vi "simple_rag_qa_chat_agent.vi"() -> ()   [LabVIEW 2020]
uses:
  <userlib>/_Soliton/LabVIEW LLM Libraries/models/llm_openai_chatmodels/llm_openai_chatmodels.lvclass
  C:/Program Files/National Instruments/LabVIEW 2020/user.lib/_Soliton/LabVIEW LLM Libraries/models/abstract_llm_base/abstract_llm_base.lvclass
  <userlib>/_Soliton/LabVIEW LLM Libraries/vectorstore/vector_qdrant/vector_qdrant.lvclass
  C:/Program Files/National Instruments/LabVIEW 2020/user.lib/_Soliton/LabVIEW LLM Libraries/vectorstore/abstract_vector_base/abstract_vector_base.lvclass
  <userlib>/_Soliton/LabVIEW LLM Libraries/models/llm_openai_embedding/llm_openai_embedding.lvclass
  <userlib>/_Soliton/LabVIEW LLM Libraries/models/llm_openai_chatmodels/Instantiate_llm_openai.vi
  <userlib>/_Soliton/LabVIEW LLM Libraries/models/llm_openai_embedding/Instantiate_llm_openai_embed.vi
  <userlib>/_Soliton/LabVIEW LLM Libraries/models/message_text/create_text_message.vi
  <userlib>/_Soliton/LabVIEW LLM Libraries/agent/agent_simple_qa/agent_simple_qa.lvclass
  <userlib>/_Soliton/LabVIEW LLM Libraries/user_interfaces/simple_html_chat_ui/simple_html_chat_ui.lvclass
  <userlib>/_Soliton/LabVIEW LLM Libraries/models/message_text/message_text.lvclass
panel:
  in  "new_message":string
  in  "send":bool
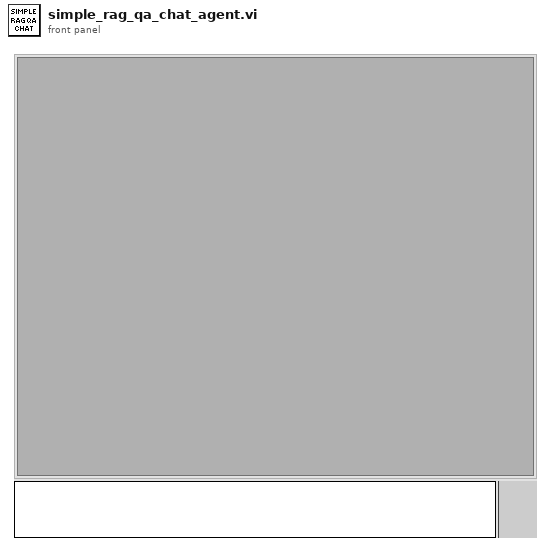
[diagram p1: front panel]
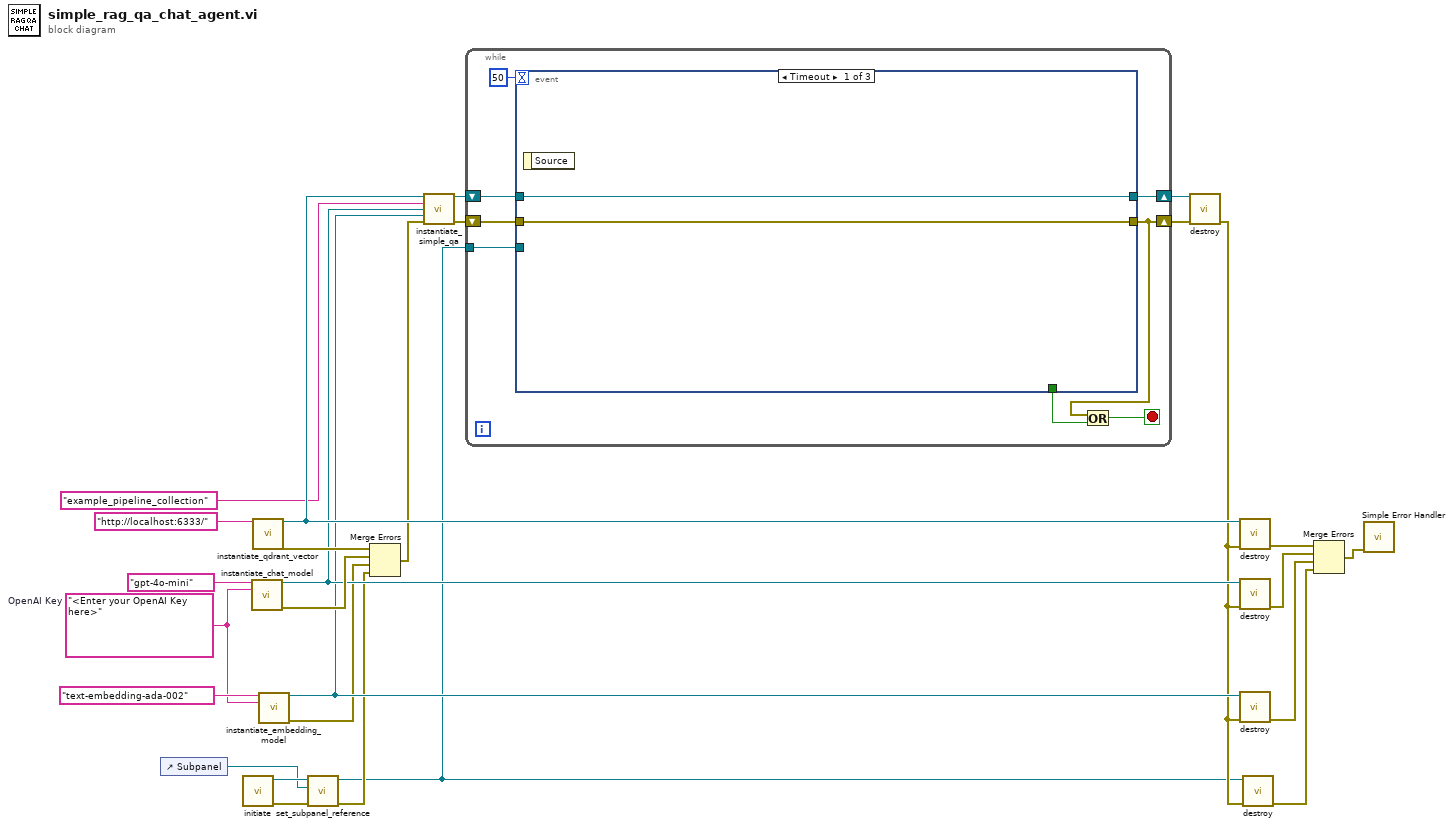
[diagram p0: block diagram]
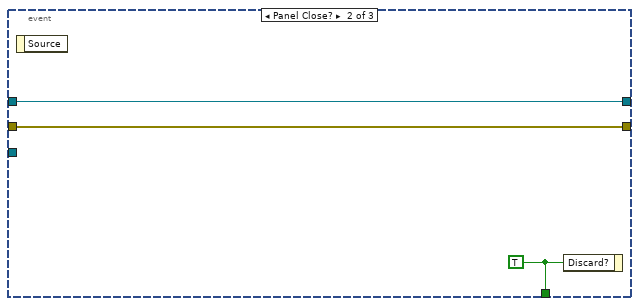
[diagram p2: hidden frame]
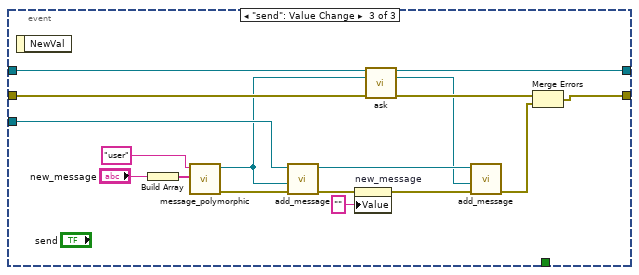
[diagram p3: hidden frame]
diagram:
  w1 = "<Enter your OpenAI Key here>"  # OpenAI Key
  n1 = control-ref of="Subpanel"() -> (w5:refnum<vi>)
  n2 = call <userlib>:"initiate.vi"() -> ("error out"=w8:errorcluster, "simple_html_chat_ui out"=w6:refnum<class "simple_html_chat_ui.lvclass">)  [unwired: 10 in]
  n3 = call-poly <userlib>:"instantiate_chat_model.vi"("model_name"="gpt-4o-mini", "openai_key"=w1) -> ("llm_openai out"=w14:refnum<class "llm_openai_chatmodels.lvclass">, "error out"=w16:errorcluster)  [unwired: 12 in]
  n4 = call <userlib>:"instantiate_qdrant_vector.vi"("host_url"="http://localhost:6333/") -> ("vector_qdrant out"=w21:refnum<class "vector_qdrant.lvclass">, "error out"=w17:errorcluster)  [unwired: 13 in]
  n5 = call-poly <userlib>:"instantiate_embedding_model.vi"("model_name"="text-embedding-ada-002", "openai_key"=w1) -> ("llm_openai_embedding out"=w11:refnum<class "llm_openai_embedding.lvclass">, "error out"=w10:errorcluster)  [unwired: 12 in]
  n6 = call <userlib>:"set_subpanel_reference.vi"("error in (no error)"=w8, "Sub Panel"=w5, "simple_html_chat_ui in"=w6) -> ("error out"=w7:errorcluster, "simple_html_chat_ui out"=w2:refnum<class "simple_html_chat_ui.lvclass">)  [unwired: 7 in]
  n7 = Merge Errors(w17, w16, w10, w7) -> (w15:errorcluster)
  n8 = call <userlib>:"instantiate_simple_qa.vi"("vectorestore"=w21, "collection_name"="example_pipeline_collection" ("host_url"), "chat_model"=w14, "embedding_model"=w11, "error in (no error)"=w15) -> ("agent_simple_qa out"=w27:refnum<class "agent_simple_qa.lvclass">, "error out"=w26:errorcluster)  [unwired: 9 in]
  n9 = while {
    shift-right: [w32] -> w25
    shift-left: w27 -> [w33]
    shift-right: [w29] -> w24
    shift-left: w26 -> [w31]
    tunnel: w2 -> [w28]
    stop <- w30 stop-if-true
    n10 = event shown="[0] Timeout" {
      selector: _ -> [_ _ _]
      dyn-events: _ -> [_ _ _]
      timeout: 50 -> [_ _ _]
      tunnel: [_ w40 _] -> w35
      tunnel: w33 -> [w36 w39 w57]
      tunnel: [w36 w39 w56] -> w32
      tunnel: w31 -> [w37 w38 w55]
      tunnel: [w37 w38 w50] -> w29
      tunnel: w28 -> [_ _ w47]
      event Timeout {
        n11 = event-data() -> ()  [unwired: 1 in, 1 out]
      }
      event Panel Close? {
        w40 = TRUE ("Discard?")
        n12 = event-data() -> ()  [unwired: 1 in, 1 out]
        n13 = event-data("Discard?"=w40) -> ()  [unwired: 1 in, 1 out]
      }
      event "send": Value Change {
        n14 = event-data() -> ()  [unwired: 1 in, 1 out]
        n15 = Build Array("new_message") -> (w51:string[])
        n16 = call-poly <userlib>:"message_polymorphic.vi"("content"=w51, "role"="user") -> ("error out"=w48:errorcluster, "message_text out"=w45:refnum<class "message_text.lvclass">)  [unwired: 8 in]
        n17 = call <userlib>:"add_message.vi"("error in (no error)"=w48, "message_text.lvclass"=w45, "simple_html_chat_ui in"=w47) -> ("error out"=w43:errorcluster, "simple_html_chat_ui out"=w46:refnum<class "simple_html_chat_ui.lvclass">)  [unwired: 7 in]
        n18 = property on="new_message" class="Str"(error in=w43, "Value"="" ("new_message")) -> (error out=w42:errorcluster)  [unwired: 1 in, 1 out]
        n19 = call-dynamic "ask.vi"("agent_simple_qa in"=w57, "message_text"=w45, "error in (no error)"=w55) -> ("agent_simple_qa out"=w56:refnum<class "agent_simple_qa.lvclass">, "message_text_response"=w44:refnum<class "message_text.lvclass">, "error out"=w54:errorcluster)  [unwired: 10 in]
        n20 = call <userlib>:"add_message.vi"("error in (no error)"=w42, "message_text.lvclass"=w44, "simple_html_chat_ui in"=w46) -> ("error out"=w49:errorcluster)  [unwired: 7 in, 1 out]
        n21 = Merge Errors(w54, w49) -> (w50:errorcluster)
      }
    }
    n22 = Or(x=w29, y=w35) -> (x .or. y?=w30:bool)
  }
  n23 = call-dynamic <userlib>:"destroy.vi"("agent_simple_qa in"=w25, "error in (no error)"=w24) -> ("error out"=w4:errorcluster)  [unwired: 12 in, 1 out]
  n24 = call-dynamic <userlib>:"destroy.vi"("vector_qdrant in"=w21, "error in (no error)"=w4) -> ("error out"=w20:errorcluster)  [unwired: 12 in, 1 out]
  n25 = call-dynamic <userlib>:"destroy.vi"("error in (no error)"=w4, "abstract_llm_base in"=w14) -> ("error out"=w19:errorcluster)  [unwired: 8 in, 1 out]
  n26 = call-dynamic <userlib>:"destroy.vi"("error in (no error)"=w4, "llm_openai_embedding in"=w11) -> ("error out"=w9:errorcluster)  [unwired: 8 in, 1 out]
  n27 = call <userlib>:"destroy.vi"("error in (no error)"=w4, "simple_html_chat_ui in"=w2) -> ("error out"=w3:errorcluster)  [unwired: 8 in, 1 out]
  n28 = Merge Errors(w20, w19, w9, w3) -> (w18:errorcluster)
  n29 = call <vilib>:"Simple Error Handler.vi"("error in (no error)"=w18) -> ()  [unwired: 4 in, 5 out]
